vi "Add Member Data.vi"(8 "error in (no error)":errorcluster, 11 "Coupled Message Scripter in":refnum<class "Coupled Message Scripter.lvclass">) -> (0 "error out":errorcluster, 3 "Coupled Message Scripter out":refnum<class "Coupled Message Scripter.lvclass">)   [LabVIEW 2020, in "Message Maker.lvlib" / "Coupled Message Scripter.lvclass"]
uses:
  Coupled Message Scripter.lvclass
  Message Scripter/Message Scripter.lvclass
  Message Maker.lvlib
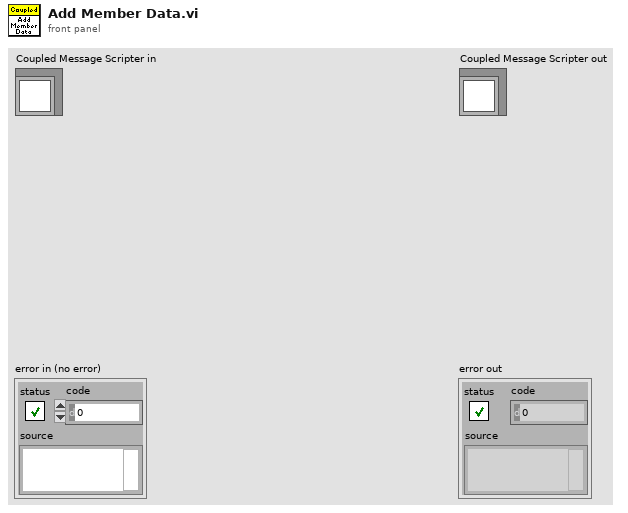
[diagram p1: front panel]
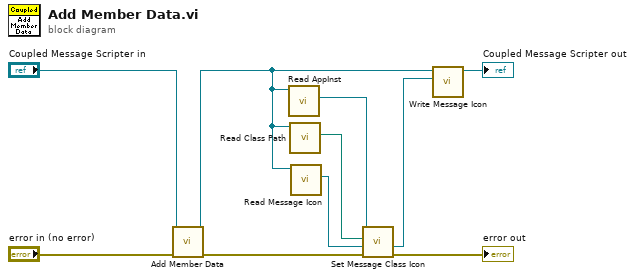
[diagram p0: block diagram]
diagram:
  n1 = call-parent "Add Member Data.vi"("error in (no error)"="error in (no error)", "Message Scripter in"="Coupled Message Scripter in") -> ("error out"=w8:errorcluster, "Message Scripter out"=w3:refnum<class "Coupled Message Scripter.lvclass">)  [unwired: 8 in]
  n2 = call "Read AppInst.vi"("Message Maker in"=w3) -> ("AppInst"=w4:refnum<vi>)  [unwired: 10 in]
  n3 = call "Read Class Path.vi"("Message Scripter in"=w3) -> ("Class Path"=w5:path)  [unwired: 10 in]
  n4 = call-dynamic "Read Message Icon.vi"("Message Scripter in"=w3) -> ("Message Icon"=w6:refnum<class "Icon.lvclass">)  [unwired: 10 in]
  n5 = call "Set Message Class Icon.vi"("error in (no error)"=w8, "Icon in"=w6, "New Class Path"=w5, "AppInst"=w4) -> ("error out"=→"error out":errorcluster, "Icon out"=w1:refnum<class "Icon.lvclass">)  [unwired: 6 in]
  n6 = call-dynamic "Write Message Icon.vi"("Message Icon"=w1, "Message Scripter in"=w3) -> ("Message Scripter out"=→"Coupled Message Scripter out":refnum<class "Coupled Message Scripter.lvclass">)  [unwired: 9 in]
